vi "Conditional Disable Structure.vi"() -> ()   [LabVIEW 2023]
doc: "Conditional Disable Structures are used to enable or disable blocks of code based on Project Symbols that are set in the Project Explorer. Project Symbol values are strings that are compared to the conditions set in the Conditional Disable Structure at run time. Code that has been disabled in this manner is not compiled or checked for errors."
panel:
  in  "Z":i32=4
  in  "Y":i32=2
  in  "X":i32=1
  out "Result":i32
  # "Overview: Demonstrates the use of a Conditional Disable Structure to execute a certain section of code based on the values of conditional symbols.\nInstructions:\n1. Make sure you have opened this VI from within Disable Structures.lvproj, and not directly from disk.\n2. Run the VI. It will run the Symbol1=True condition on the block diagram.\n3. In the Project Explorer window, right-click the top-level project entry in the Items tree and select Properties.\n4. On the Conditional Disable Symbols page, change the value of Symbol1 to \"False\" and click OK.\n5. Run the VI again. It will run a different condition on the block diagram, even though the code did not change."
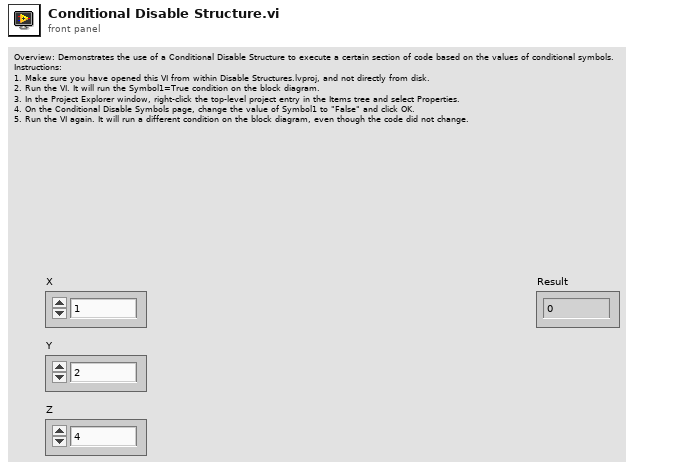
[diagram p1: front panel]
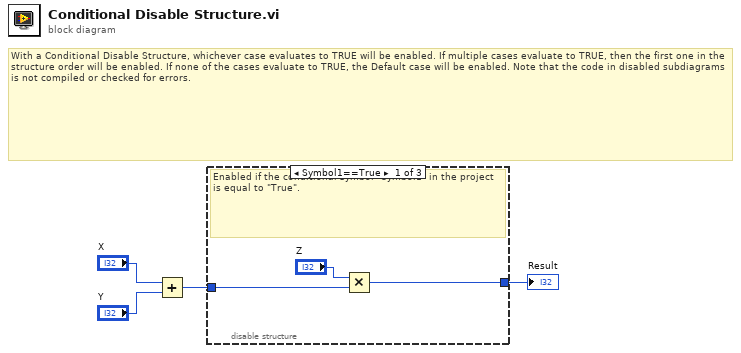
[diagram p0: block diagram]
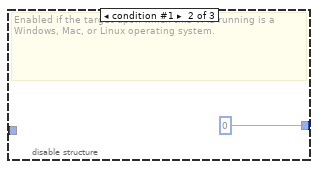
[diagram p2: hidden frame]
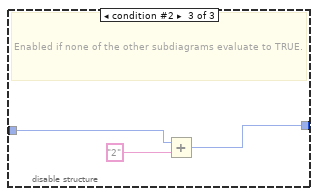
[diagram p3: hidden frame]
diagram:
  # "With a Conditional Disable Structure, whichever case evaluates to TRUE will be enabled. If multiple cases evaluate to TRUE, then the first one in the structure order will be enabled. If none of the cases evaluate to TRUE, the Default case will be enabled. Note that the code in disabled subdiagrams is not compiled or checked for errors."
  n1 = Add(x="X", y="Y") -> (x+y=w2:i32)
  n2 = disable-structure shown="Symbol1==True" {
    disable-tunnel: w2 -> [w7 _ w11]
    disable-tunnel: [w6 0 w10] -> w1
    frame condition #0 (active) {
      # "Enabled if the conditional symbol \"Symbol1\" in the project is equal to \"True\"."
      n3 = Multiply(x="Z", y=w7) -> (x*y=w6:i32)
    }
    frame condition #1 {
      # "Enabled if the target upon which this VI is running is a Windows, Mac, or Linux operating system."
    }
    frame condition #2 {
      # "Enabled if none of the other subdiagrams evaluate to TRUE."
      n4 = Add(x=w11, y="2") -> (x+y=w10:i32)
    }
  }
  "Result" <- w1
